vi "return.vi"(10 "Colors and Directions":enum16{"Zero", "Right", "Front", "Left"}[](array[ring])=[enum."Zero", enum."Zero", enum."Zero", enum."Zero", enum."Zero", enum."Zero"]) -> (1 "Colors and Directions 2":enum16{"Zero", "Right", "Front", "Left"}[](array[ring])=[enum."Zero", enum."Zero", enum."Zero", enum."Zero", enum."Zero", enum."Zero"])   [LabVIEW 2016]
uses:
  <vilib>/NXT/Subs/ColorSensorColors.ctl
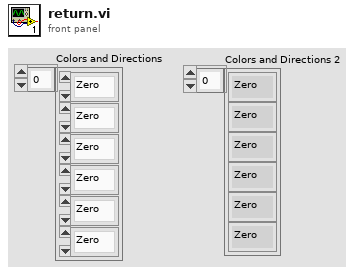
[diagram p1: front panel]
types:
  T1 = typedef "ColorSensorColors.ctl" = enum16{"No Color", "Black", "Blue", "Green", "Yellow", "Red", "White", "Brown"}
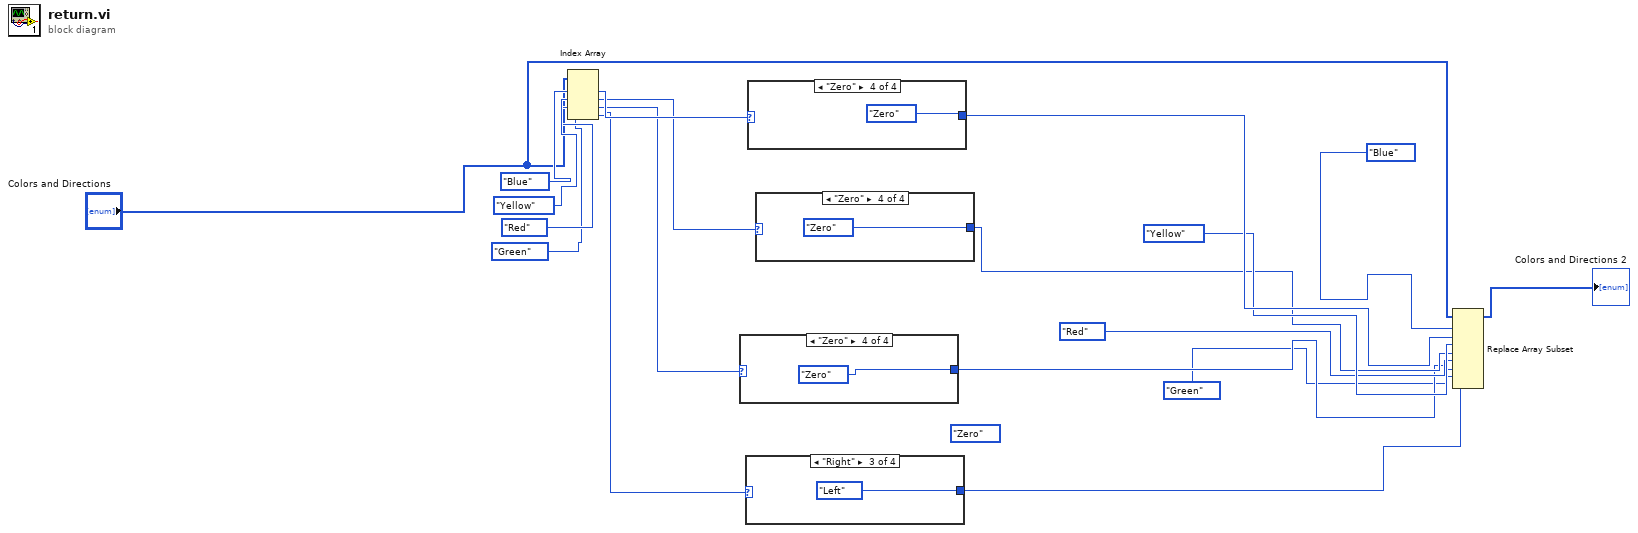
[diagram p0: block diagram]
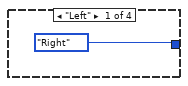
[diagram p2: hidden frame]
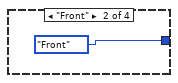
[diagram p3: hidden frame]
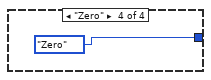
[diagram p4: hidden frame]
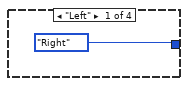
[diagram p5: hidden frame]
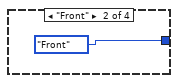
[diagram p6: hidden frame]
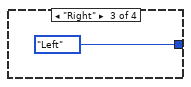
[diagram p7: hidden frame]
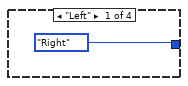
[diagram p8: hidden frame]
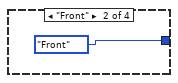
[diagram p9: hidden frame]
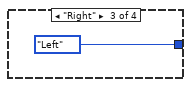
[diagram p10: hidden frame]
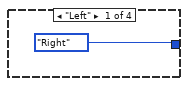
[diagram p11: hidden frame]
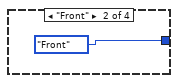
[diagram p12: hidden frame]
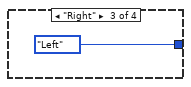
[diagram p13: hidden frame]
diagram:
  (unwired) enum16{"Zero", "Right", "Front", "Left"}."Zero" ("Direction")
  n1 = Index Array(array="Colors and Directions", index #1=ColorSensorColors."Blue" ("Detected Color"), index #2=ColorSensorColors."Yellow" ("Detected Color"), index #3=ColorSensorColors."Red" ("Detected Color"), index #4=ColorSensorColors."Green" ("Detected Color")) -> (element #1=w5:enum16{"Zero", "Right", "Front", "Left"}, element #2=w4:enum16{"Zero", "Right", "Front", "Left"}, element #3=w3:enum16{"Zero", "Right", "Front", "Left"}, element #4=w2:enum16{"Zero", "Right", "Front", "Left"})
  n2 = case shown="\"Zero\"" w3 {
    tunnel: [enum16{"Zero", "Right", "Front", "Left"}."Right" ("Direction") enum16{"Zero", "Right", "Front", "Left"}."Front" ("Direction") enum16{"Zero", "Right", "Front", "Left"}."Left" ("Direction") enum16{"Zero", "Right", "Front", "Left"}."Zero" ("Direction")] -> w13
    frame "Left" {
    }
    frame "Front" {
    }
    frame "Right" {
    }
    frame "Zero" {
    }
  }
  n3 = case shown="\"Right\"" w2 {
    tunnel: [enum16{"Zero", "Right", "Front", "Left"}."Right" ("Direction") enum16{"Zero", "Right", "Front", "Left"}."Front" ("Direction") enum16{"Zero", "Right", "Front", "Left"}."Left" ("Direction") enum16{"Zero", "Right", "Front", "Left"}."Zero" ("Direction")] -> w11
    frame "Left" {
    }
    frame "Front" {
    }
    frame "Right" {
    }
    frame "Zero" {
    }
  }
  n4 = case shown="\"Zero\"" w5 {
    tunnel: [enum16{"Zero", "Right", "Front", "Left"}."Right" ("Direction") enum16{"Zero", "Right", "Front", "Left"}."Front" ("Direction") enum16{"Zero", "Right", "Front", "Left"}."Left" ("Direction") enum16{"Zero", "Right", "Front", "Left"}."Zero" ("Direction")] -> w17
    frame "Left" {
    }
    frame "Front" {
    }
    frame "Right" {
    }
    frame "Zero" {
    }
  }
  n5 = case shown="\"Zero\"" w4 {
    tunnel: [enum16{"Zero", "Right", "Front", "Left"}."Right" ("Direction") enum16{"Zero", "Right", "Front", "Left"}."Front" ("Direction") enum16{"Zero", "Right", "Front", "Left"}."Left" ("Direction") enum16{"Zero", "Right", "Front", "Left"}."Zero" ("Direction")] -> w15
    frame "Left" {
    }
    frame "Front" {
    }
    frame "Right" {
    }
    frame "Zero" {
    }
  }
  n6 = Replace Array Subset(array="Colors and Directions", new element #1=w17, index #1=ColorSensorColors."Blue" ("Detected Color"), new element #2=w15, index #2=ColorSensorColors."Yellow" ("Detected Color"), new element #3=w13, index #3=ColorSensorColors."Red" ("Detected Color"), new element #4=w11, index #4=ColorSensorColors."Green" ("Detected Color")) -> (→"Colors and Directions 2":enum16{"Zero", "Right", "Front", "Left"}[])
